vi "Finish.vi"(4 "error in":errorcluster) -> (0 "error out":errorcluster)   [LabVIEW 2016]
doc: "This VI is called just before exiting. It is expected to close I/O refnum, save collected data, etc."
uses:
  <vilib>/Rock Robotics/WPI/Utilities/WPI_GetSetVariantRefNum.vi
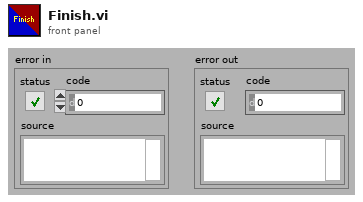
[diagram p1: front panel]
types:
  T1 = typedef "WPI_JoystickDevRef.ctl" = cluster{"Device":T2}
  T2 = typedef "WPI_JoystickDeviceEnum.ctl" = enum16{"USB 0", "USB 1", "USB 2", "USB 3", "USB 4", "USB 5"}
  T3 = typedef "WPI_RobotDriveDevRef.ctl" = cluster{"DevStatus":errorcluster, "Motors[]":T4[], "Square Inputs":bool, "Max Output":dbl}
  T4 = typedef "WPI_MotorControlDeviceRef.ctl" = cluster{"DeviceStatus":errorcluster, "Type":T5, "PWM":cluster{"PWM Channel":T6, "DeadBand":T7}, "CAN":cluster{"Device Number":u8, "SetOutput VI Ref":variant, "GetOutput VI Ref":variant, "Enable VI Ref":variant, "Disable VI Ref":variant, "Data":variant}, "Invert":bool}
  T5 = typedef "WPI_MotorControlType.ctl" = enum16{"PWM", "CAN"}
  T6 = typedef "FPGA_DIOPWMChannel.ctl" = enum8{"PWM 0", "PWM 1", "PWM 2", "PWM 3", "PWM 4", "PWM 5", "PWM 6", "PWM 7", "PWM 8", "PWM 9", "PWM MXP 0", "PWM MXP 1", "PWM MXP 2", "PWM MXP 3", "PWM MXP 4", "PWM MXP 5", "PWM MXP 6", "PWM MXP 7", "PWM MXP 8", "PWM MXP 9", "Invalid"}
  T7 = typedef "WPI_PWMDeadband.ctl" = cluster{"Name":string, "maxPositivePwm":i32, "minPositivePwm":i32, "centerPwm":i32, "maxNegativePwm":i32, "minNegativePwm":i32, "angularRange":u16}
  T8 = typedef "WPI_EncoderDevRef.ctl" = cluster{"DevStatus":errorcluster, "EncoderIndex":T9, "CounterIndex":T10, "DistancePerCount":dbl, "Decoding Type":T11}
  T9 = typedef "FPGA_EncoderIdx.ctl" = enum8{"Enc 0", "Enc 1", "Enc 2", "Enc 3", "Enc 4", "Enc 5", "Enc 6", "Enc 7", "Invalid"}
  T10 = typedef "FPGA_CounterCtrSystemIndex.ctl" = enum8{"Ctr 0", "Ctr 1", "Ctr 2", "Ctr 3", "Ctr 4", "Ctr 5", "Ctr 6", "Ctr 7", "Invalid"}
  T11 = typedef "WPI_EncoderType.ctl" = enum16{"1x", "2x", "4x"}
  T12 = typedef "WPI_GyroDevRef.ctl" = cluster{"DevStatus":errorcluster, "Analog Channel":T13, "Offset":dbl, "Gain (VoltsPerDegree/Second)":dbl, "Gyro Type":enum16{"Analog", "XRS450"}, "Handle":i32, "SPI Bus":T14, "Device Found":bool, "Sample Rate":dbl, "Calibrate On Open":bool}
  T13 = typedef "FPGA_AIChannel.ctl" = enum8{"AI 0", "AI 1", "AI 2", "AI 3", "AI MXP 0", "AI MXP 1", "AI MXP 2", "AI MXP 3", "Invalid"}
  T14 = typedef "spi_bus.ctl" = enum16{"SPI On-Board, CS0", "SPI On-Board, CS1", "SPI On-Board, CS2", "SPI On-Board, CS3", "SPI MXP", "Invalid"}
  T15 = typedef "WPI_AccelerometerDevRef.ctl" = cluster{"DevStatus":errorcluster, "Scaling":T16, "Analog Channels":T17, "I2C Bus":T18, "SPI Bus":T14, "Accel Range":T19, "ADXL Axes":T20, "Handle":i32, "Device Address":u8, "Accel Type":enum16{"Analog", "ADXL345 I2C", "ADXL345 SPI", "Internal", "ADXL362 SPI"}}
  T16 = typedef "WPI_AccelerometerScaling.ctl" = cluster{"Gain (VoltsPerG)":dbl, "Center Voltage":dbl}
  T17 = typedef "WPI_AccelerometerAnalogChannels.ctl" = cluster{"X-Axis":T13, "Y-Axis":T13, "Z-Axis":T13}
  T18 = typedef "i2c_bus.ctl" = enum16{"I2C On-Board", "I2C MXP", "Invalid"}
  T19 = typedef "ADXL345 Range.ctl" = u8
  T20 = typedef "WPI_AccelerometerADXL345 Axes.ctl" = cluster{"X-Axis":bool, "Y-Axis":bool, "Z-Axis":bool}
  T21 = typedef "WPI_AnalogChannelDevRef.ctl" = cluster{"DevStatus":errorcluster, "Analog Channel":T13}
  T22 = typedef "WPI_DigitalInputDevRef.ctl" = cluster{"DevStatus":errorcluster, "DIO Channel":T23}
  T23 = typedef "FPGA_DIOChannel.ctl" = enum8{"DIO 0", "DIO 1", "DIO 2", "DIO 3", "DIO 4", "DIO 5", "DIO 6", "DIO 7", "DIO 8", "DIO 9", "DIO MXP 0", "DIO MXP 1", "DIO MXP 2", "DIO MXP 3", "DIO MXP 4", "DIO MXP 5", "DIO MXP 6", "DIO MXP 7", "DIO MXP 8", "DIO MXP 9", "DIO MXP 10", "DIO MXP 11", "DIO MXP 12", "DIO MXP 13", "DIO MXP 14", "DIO MXP 15", "SPI Port CS1", "SPI Port CS2", "SPI Port CS3", "SPI Port MISO", "SPI Port MOSI", "Invalid"}
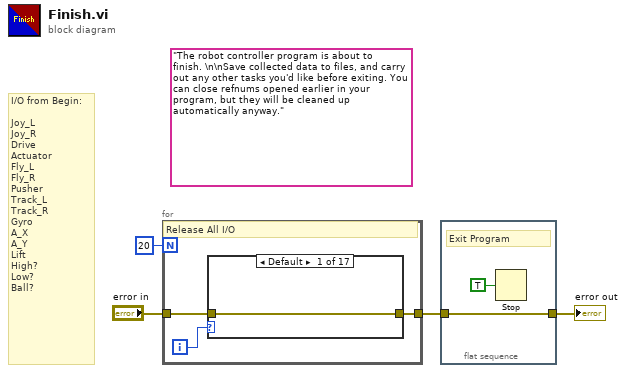
[diagram p0: block diagram]
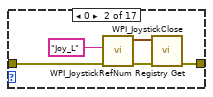
[diagram p2: hidden frame]
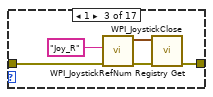
[diagram p3: hidden frame]
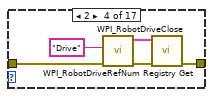
[diagram p4: hidden frame]
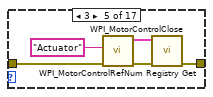
[diagram p5: hidden frame]
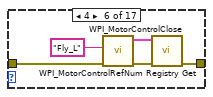
[diagram p6: hidden frame]
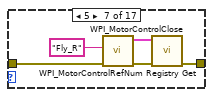
[diagram p7: hidden frame]
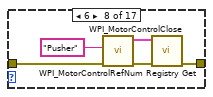
[diagram p8: hidden frame]
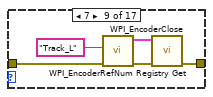
[diagram p9: hidden frame]
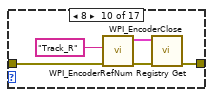
[diagram p10: hidden frame]
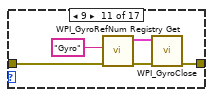
[diagram p11: hidden frame]
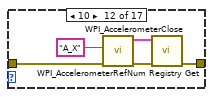
[diagram p12: hidden frame]
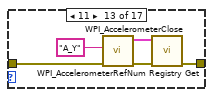
[diagram p13: hidden frame]
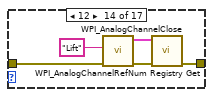
[diagram p14: hidden frame]
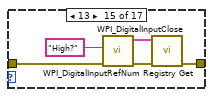
[diagram p15: hidden frame]
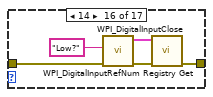
[diagram p16: hidden frame]
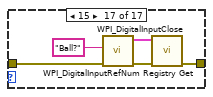
[diagram p17: hidden frame]
diagram:
  (unwired) "The robot controller program is about to finish. \n\nSave collected data to files, and carry out any other tasks you'd like before exiting. You can close refnums opened earlier in your program, but they will be cleaned up automatically anyway."
  # "I/O from Begin:\n\nJoy_L\nJoy_R\nDrive\nActuator\nFly_L\nFly_R\nPusher\nTrack_L\nTrack_R\nGyro\nA_X\nA_Y\nLift\nHigh?\nLow?\nBall?"
  n1 = for {
    N: 20 -> [_]
    tunnel: "error in" -> [w6]
    tunnel: [w5] -> w1
    i -> [w7]
    # "Release All I/O"
    n2 = case shown="Default" w7 {
      tunnel: w6 -> [w8 w10 w14 w20 w25 w30 w35 w40 w45 w50 w55 w60 w65 w70 w75 w80 w85]
      tunnel: [w8 w9 w13 w17 w23 w28 w33 w38 w43 w48 w53 w58 w63 w68 w73 w78 w83] -> w5
      frame Default {
      }
      frame 0 {
        n3 = call <vilib>:"WPI_JoystickRefNum Registry Get.vi"("error in (no error)"=w10, "refnum name"="Joy_L") -> ("error out"=w9:errorcluster, "JoystickDevRef"=w11:T1)  [unwired: 8 out]
        n4 = call <vilib>:"WPI_JoystickClose.vi"("JoystickDevRef"=w11) -> ()  [unwired: 11 out]
      }
      frame 1 {
        n5 = call <vilib>:"WPI_JoystickRefNum Registry Get.vi"("error in (no error)"=w14, "refnum name"="Joy_R") -> ("error out"=w13:errorcluster, "JoystickDevRef"=w15:T1)  [unwired: 8 out]
        n6 = call <vilib>:"WPI_JoystickClose.vi"("JoystickDevRef"=w15) -> ()  [unwired: 11 out]
      }
      frame 2 {
        n7 = call <vilib>:"WPI_RobotDriveRefNum Registry Get.vi"("error in (no error)"=w20, "refnum name"="Drive") -> ("error out"=w18:errorcluster, "RobotDriveDevRef"=w19:T3)  [unwired: 8 in]
        n8 = call <vilib>:"WPI_RobotDriveClose.vi"("error in (no error)"=w18, "RobotDriveDevRef"=w19) -> ("error out"=w17:errorcluster)  [unwired: 9 in]
      }
      frame 3 {
        n9 = call <vilib>:"WPI_MotorControlRefNum Registry Get.vi"("error in (no error)"=w25, "refnum name"="Actuator") -> ("error out"=w24:errorcluster, "MotorControlDevRef"=w22:T4)  [unwired: 8 in]
        n10 = call <vilib>:"WPI_MotorControlClose.vi"("error in"=w24, "MotorControlDevRef"=w22) -> ("error out"=w23:errorcluster)  [unwired: 9 in]
      }
      frame 4 {
        n11 = call <vilib>:"WPI_MotorControlRefNum Registry Get.vi"("error in (no error)"=w30, "refnum name"="Fly_L") -> ("error out"=w29:errorcluster, "MotorControlDevRef"=w27:T4)  [unwired: 8 in]
        n12 = call <vilib>:"WPI_MotorControlClose.vi"("error in"=w29, "MotorControlDevRef"=w27) -> ("error out"=w28:errorcluster)  [unwired: 9 in]
      }
      frame 5 {
        n13 = call <vilib>:"WPI_MotorControlRefNum Registry Get.vi"("error in (no error)"=w35, "refnum name"="Fly_R") -> ("error out"=w34:errorcluster, "MotorControlDevRef"=w32:T4)  [unwired: 8 in]
        n14 = call <vilib>:"WPI_MotorControlClose.vi"("error in"=w34, "MotorControlDevRef"=w32) -> ("error out"=w33:errorcluster)  [unwired: 9 in]
      }
      frame 6 {
        n15 = call <vilib>:"WPI_MotorControlRefNum Registry Get.vi"("error in (no error)"=w40, "refnum name"="Pusher") -> ("error out"=w39:errorcluster, "MotorControlDevRef"=w37:T4)  [unwired: 8 in]
        n16 = call <vilib>:"WPI_MotorControlClose.vi"("error in"=w39, "MotorControlDevRef"=w37) -> ("error out"=w38:errorcluster)  [unwired: 9 in]
      }
      frame 7 {
        n17 = call <vilib>:"WPI_EncoderRefNum Registry Get.vi"("error in (no error)"=w45, "refnum name"="Track_L") -> ("error out"=w44:errorcluster, "EncoderDevRef"=w42:T8)  [unwired: 8 in]
        n18 = call <vilib>:"WPI_EncoderClose.vi"("error in (no error)"=w44, "EncoderDevRef"=w42) -> ("error out"=w43:errorcluster)  [unwired: 9 in]
      }
      frame 8 {
        n19 = call <vilib>:"WPI_EncoderRefNum Registry Get.vi"("error in (no error)"=w50, "refnum name"="Track_R") -> ("error out"=w49:errorcluster, "EncoderDevRef"=w47:T8)  [unwired: 8 in]
        n20 = call <vilib>:"WPI_EncoderClose.vi"("error in (no error)"=w49, "EncoderDevRef"=w47) -> ("error out"=w48:errorcluster)  [unwired: 9 in]
      }
      frame 9 {
        n21 = call <vilib>:"WPI_GyroRefNum Registry Get.vi"("error in (no error)"=w55, "refnum name"="Gyro") -> ("error out"=w54:errorcluster, "GyroDevRef"=w52:T12)  [unwired: 8 in]
        n22 = call <vilib>:"WPI_GyroClose.vi"("error in"=w54, "GyroDevRef"=w52) -> ("error out"=w53:errorcluster)  [unwired: 9 in]
      }
      frame 10 {
        n23 = call <vilib>:"WPI_AccelerometerRefNum Registry Get.vi"("error in (no error)"=w60, "refnum name"="A_X") -> ("error out"=w59:errorcluster, "AccelerometerDevRef"=w57:T15)  [unwired: 8 in]
        n24 = call <vilib>:"WPI_AccelerometerClose.vi"("error in"=w59, "AccelerometerDevRef"=w57) -> ("error out"=w58:errorcluster)  [unwired: 9 in]
      }
      frame 11 {
        n25 = call <vilib>:"WPI_AccelerometerRefNum Registry Get.vi"("error in (no error)"=w65, "refnum name"="A_Y") -> ("error out"=w64:errorcluster, "AccelerometerDevRef"=w62:T15)  [unwired: 8 in]
        n26 = call <vilib>:"WPI_AccelerometerClose.vi"("error in"=w64, "AccelerometerDevRef"=w62) -> ("error out"=w63:errorcluster)  [unwired: 9 in]
      }
      frame 12 {
        n27 = call <vilib>:"WPI_AnalogChannelRefNum Registry Get.vi"("error in (no error)"=w70, "refnum name"="Lift") -> ("error out"=w69:errorcluster, "AIDeviceRef"=w67:T21)  [unwired: 8 in]
        n28 = call <vilib>:"WPI_AnalogChannelClose.vi"("error in (no error)"=w69, "AIDeviceRef"=w67) -> ("error out"=w68:errorcluster)  [unwired: 9 in]
      }
      frame 13 {
        n29 = call <vilib>:"WPI_DigitalInputRefNum Registry Get.vi"("error in (no error)"=w75, "refnum name"="High?") -> ("error out"=w74:errorcluster, "DigitalInputDevRef"=w72:T22)  [unwired: 8 in]
        n30 = call <vilib>:"WPI_DigitalInputClose.vi"("error in (no error)"=w74, "DigitalInputDevRef"=w72) -> ("error out"=w73:errorcluster)  [unwired: 9 in]
      }
      frame 14 {
        n31 = call <vilib>:"WPI_DigitalInputRefNum Registry Get.vi"("error in (no error)"=w80, "refnum name"="Low?") -> ("error out"=w79:errorcluster, "DigitalInputDevRef"=w77:T22)  [unwired: 8 in]
        n32 = call <vilib>:"WPI_DigitalInputClose.vi"("error in (no error)"=w79, "DigitalInputDevRef"=w77) -> ("error out"=w78:errorcluster)  [unwired: 9 in]
      }
      frame 15 {
        n33 = call <vilib>:"WPI_DigitalInputRefNum Registry Get.vi"("error in (no error)"=w85, "refnum name"="Ball?") -> ("error out"=w84:errorcluster, "DigitalInputDevRef"=w82:T22)  [unwired: 8 in]
        n34 = call <vilib>:"WPI_DigitalInputClose.vi"("error in (no error)"=w84, "DigitalInputDevRef"=w82) -> ("error out"=w83:errorcluster)  [unwired: 9 in]
      }
    }
  }
  n35 = flat-sequence {
    tunnel: [w87] -> w2
    tunnel: w1 -> [w87]
    frame #0 {
      # "Exit Program"
      n36 = Stop(stop? (T)=TRUE ("Quit")) -> ()
    }
  }
  "error out" <- w2
